vi "Main.vi"(11 "Module Admin":refnum<class "Delacor_lib_QMH_Module Admin.lvclass">) -> ()   [LabVIEW 2024, in "File IO.lvlib"]
doc: "This template is based off of the Queued Message Handler design pattern and the Queued Message Handler project template that ships with LabVIEW.\n\nThe main difference is that the queue is private to this module and communication between modules is performed via Broadcast and Request events.\n\nRequest events are wrapped in public API methods and are handled in the Event Handling Loop (EHL) of this VI. Any module can register for Broadcast events sent by this module. The EHL generates messages based on user interface actions.\n\nThe Message Handling Loop (MHL) processes messages generated by the EHL, or by other messages. The messages are string values, so new messages can be added easily to the Message Cases case structure in the MHL. Each message cluster can also provide an optional value for Message Data, which is a variant that can be converted to whatever message-specific data is required.\n_____\nBased on DQMH Project Template 7.0.1.1316."
uses:
  File IO.lvlib
  <vilib>/Delacor/Delacor QMH/Libraries/Module Admin_class/Delacor_lib_QMH_Module Admin.lvclass
  Module Data--cluster.ctl
  <vilib>/Delacor/Delacor QMH/Libraries/Message Queue_class/Delacor_lib_QMH_Message Queue.lvclass/Delacor_lib_QMH_Message Queue.ctl
  Stop Argument--cluster.ctl
  <vilib>/Delacor/Delacor QMH/Libraries/Module Admin_class/Delacor_lib_QMH_Module Admin.lvclass/Delacor_lib_QMH_Module Admin.ctl
  Start Log Argument--cluster.ctl
  <vilib>/Utility/miscctls.llb/LVPointTypeDef.ctl
  <vilib>/Delacor/Delacor QMH/Libraries/Message Queue_class/Delacor_lib_QMH_Enqueue Message (Single).vi
  <vilib>/Delacor/Delacor QMH/Libraries/Module Admin_class/Delacor_lib_QMH_Get External Launch.vi
  <vilib>/Delacor/Delacor QMH/Libraries/Message Queue_class/Delacor_lib_QMH_Message Queue.lvclass
  Write Argument--cluster.ctl
  <vilib>/Utility/sysdir.llb/System Directory Type.ctl
panel:
  out "File Created":bool=TRUE
  out "error out":errorcluster
  out "Status":string
  in  "Simulate MHL Error":bool
  in  "Simulate EHL Error":bool
  # "Other processes communicate with this Module via its Public API (wrappers for its Request Events).\n\nThis Module communicates with other processes via its Broadcast Events.\nAny process that wants to receive these messages can register for this module's Broadcast events."
  # "This template is for the DQMH framework. See the block diagram for more information on how to use this template."
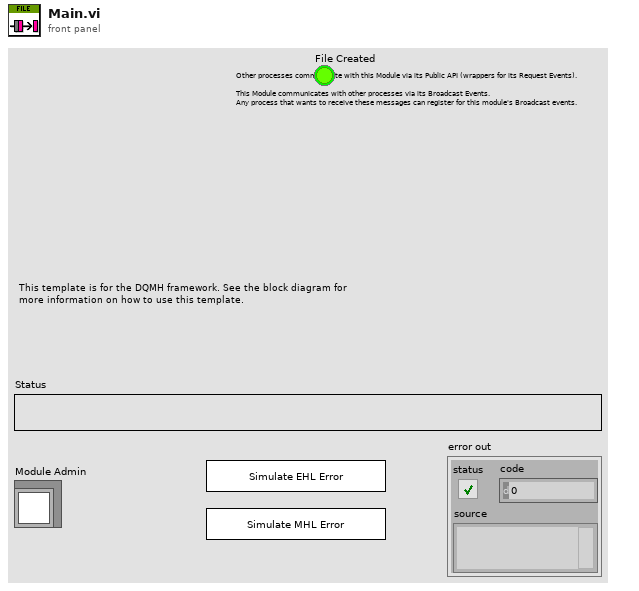
[diagram p1: front panel]
types:
  T1 = typedef "File IO.lvlib/Request Events--cluster.ctl" = cluster{"Stop Module":refnum<user-event>, "Show Panel":refnum<user-event>, "Hide Panel":refnum<user-event>, "Get Module Execution Status":refnum<user-event>, "Show Diagram":refnum<user-event>, "Start Log":refnum<user-event>, "Write":refnum<user-event>}
  T2 = typedef "File IO.lvlib/Module Data--cluster.ctl" = cluster{"Status":string, "LogFilePath":path}
  T3 = enum32{"invalid lock state", "Not Locked", "Locked (No Password)", "Password-protected"}
  T4 = typedef "File IO.lvlib/Stop Argument--cluster.ctl" = cluster{"Origin":string, "Exit via Stop Module Req?":bool, "Wait for Module to stop?":bool}
  T5 = typedef "File IO.lvlib/Start Log Argument--cluster.ctl" = cluster{"Boolean":bool}
  T6 = typedef "File IO.lvlib/Write Argument--cluster.ctl" = cluster{"Write String":string}
  T7 = typedef "LVPointTypeDef.ctl" = cluster{"Horizontal":i16, "Vertical":i16}
  T8 = enum32{"Invalid", "Standard", "Closed", "Hidden", "Minimized", "Maximized"}
  T9 = enum16{"open", "replace", "create", "open or create", "replace or create", "replace or create with confirmation"}
  T10 = typedef "System Directory Type.ctl" = i32
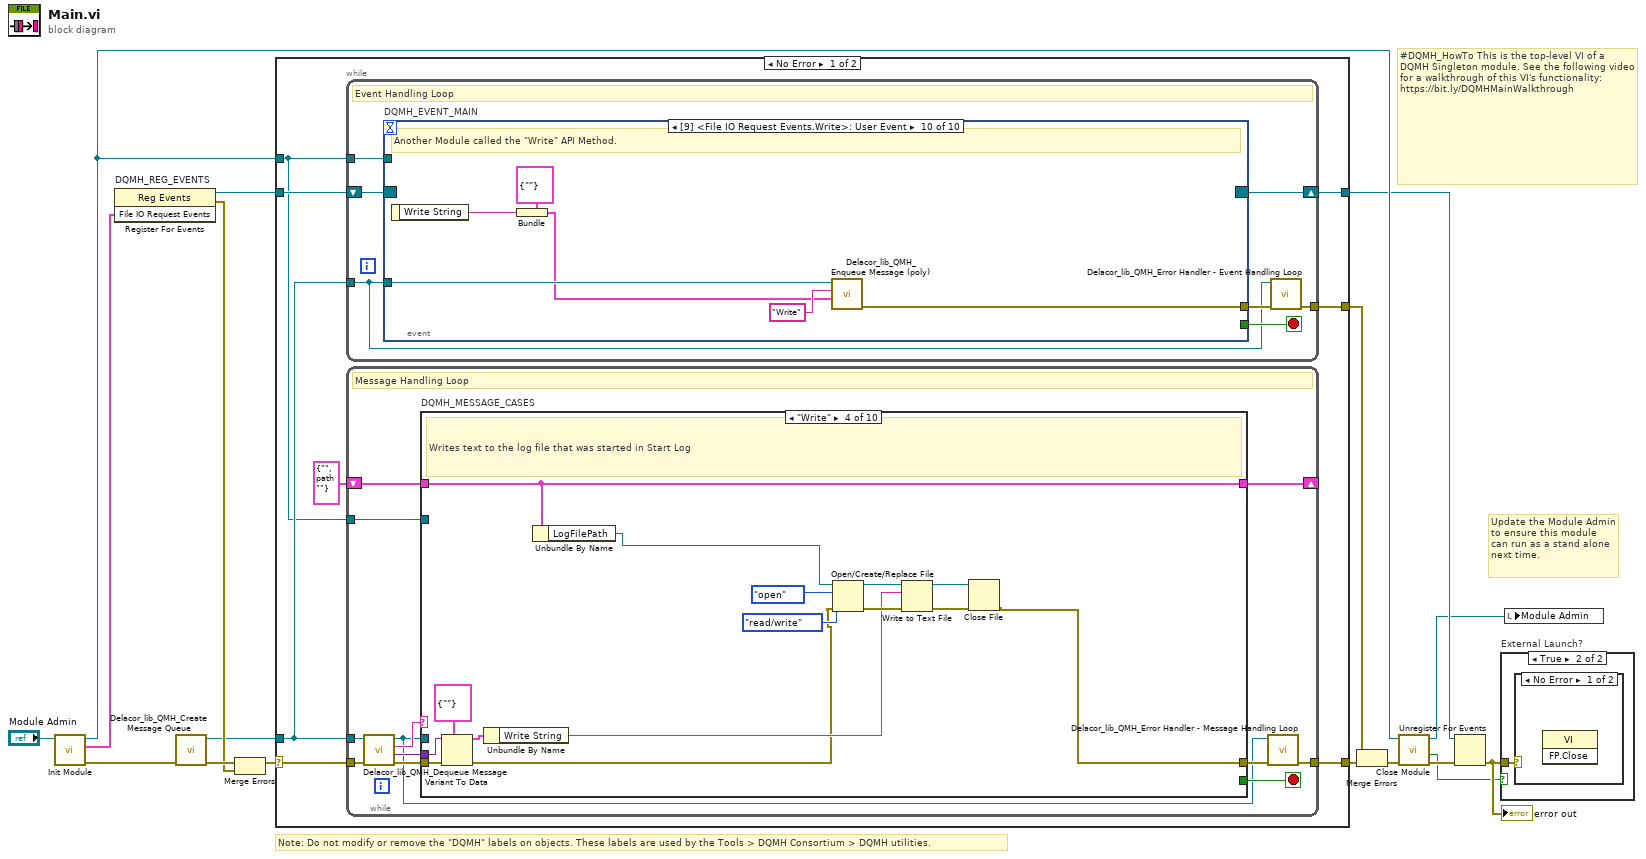
[diagram p0: block diagram]
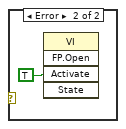
[diagram p3: hidden frame]
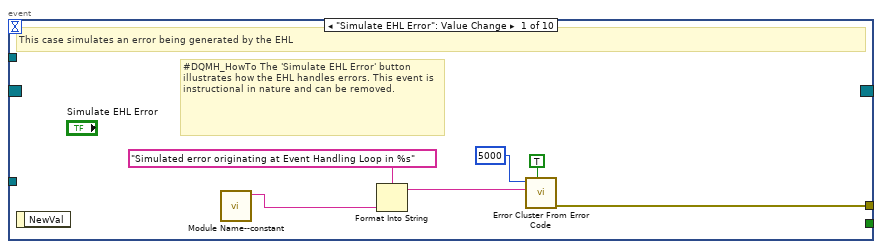
[diagram p4: hidden frame]
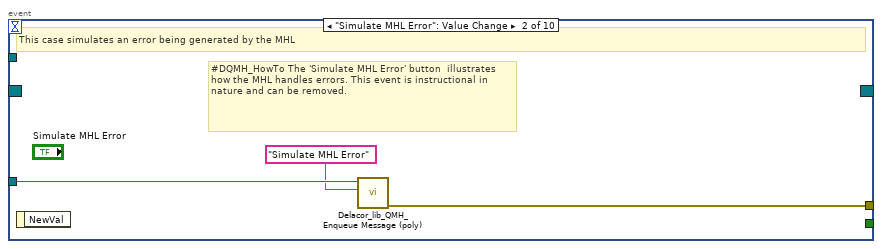
[diagram p5: hidden frame]
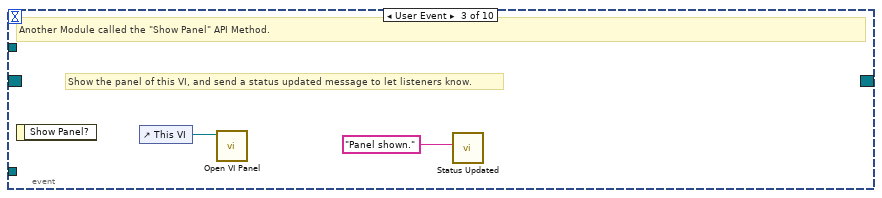
[diagram p6: hidden frame]
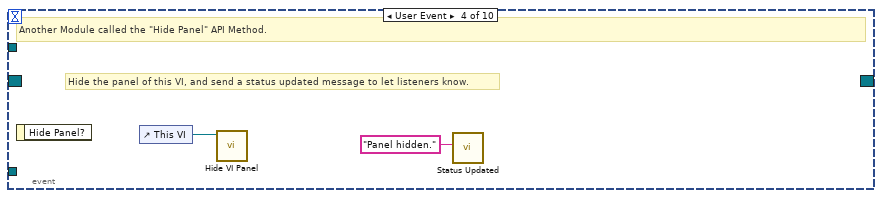
[diagram p7: hidden frame]
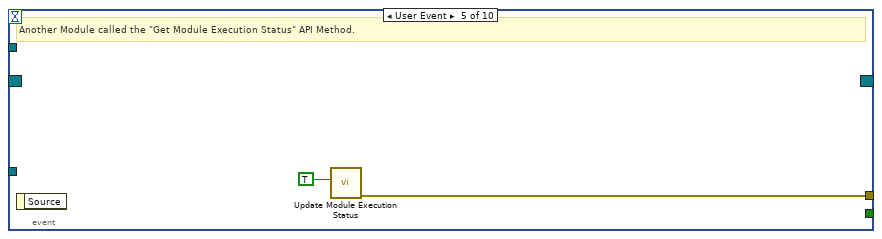
[diagram p8: hidden frame]
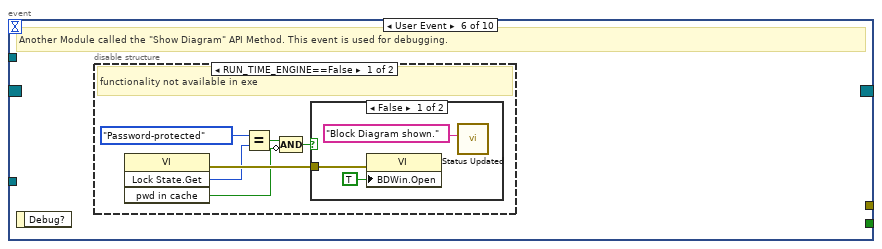
[diagram p9: hidden frame]
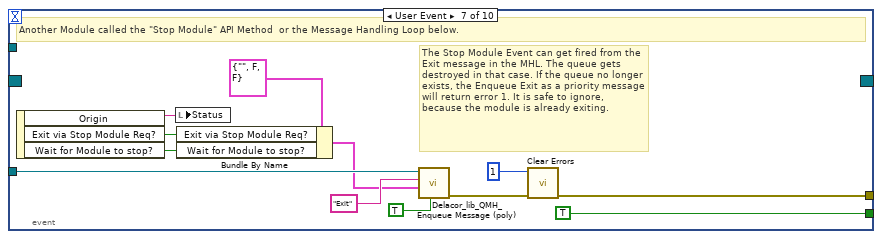
[diagram p12: hidden frame]
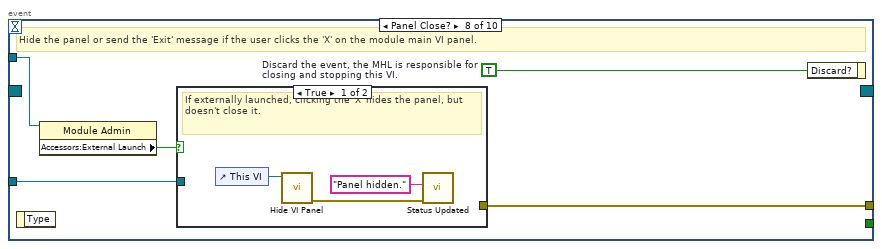
[diagram p13: hidden frame]
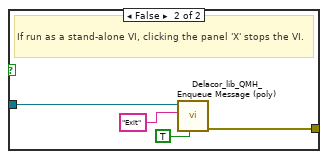
[diagram p14: hidden frame]
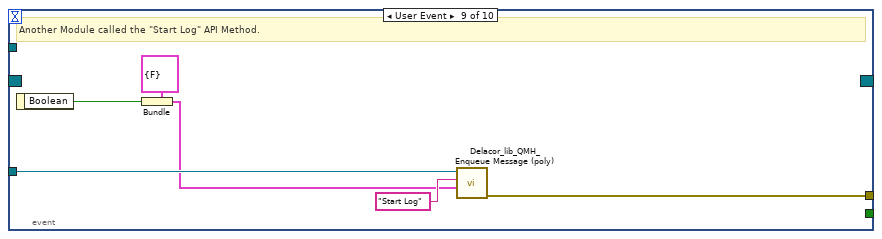
[diagram p15: hidden frame]
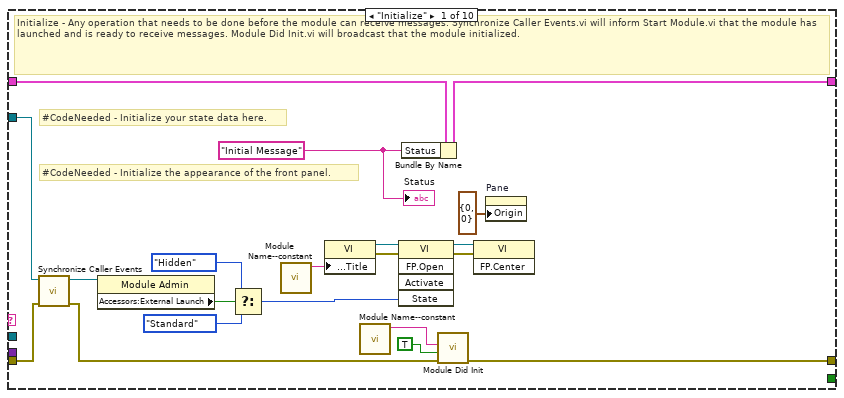
[diagram p16: hidden frame]
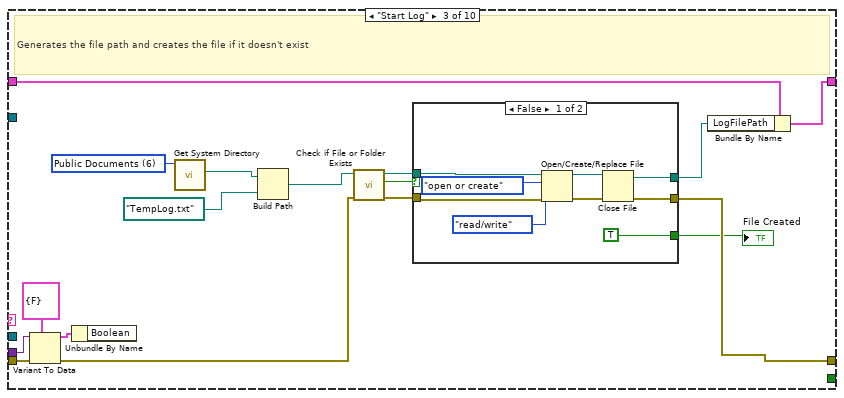
[diagram p18: hidden frame]
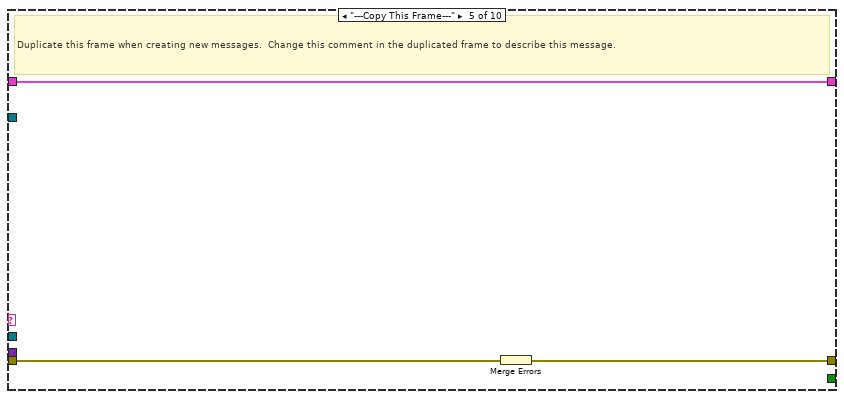
[diagram p20: hidden frame]
diagram:
  # "#DQMH_HowTo This is the top-level VI of a DQMH Singleton module. See the following video for a walkthrough of this VI's functionality: https://bit.ly/DQMHMainWalkthrough"
  # "Note: Do not modify or remove the \"DQMH\" labels on objects. These labels are used by the Tools > DQMH Consortium > DQMH utilities."
  # "Update the Module Admin to ensure this module can run as a stand alone next time."
  n1 = call "Init Module.vi"("Singleton Module Admin in"="Module Admin") -> ("error out"=w16:errorcluster, "File IO Request Events"=w5:T1, "Singleton Module Admin out"=w8:refnum<class "Delacor_lib_QMH_Module Admin.lvclass">)  [unwired: 8 in]
  n2 = register-events "DQMH_REG_EVENTS"(w5) -> (reference out=w6:refnum<event-registration>, error out=w9:errorcluster)  [unwired: 2 in]
  n3 = call <vilib>:"Delacor_lib_QMH_Create Message Queue.vi"("error in"=w16) -> ("error out"=w11:errorcluster, "Message Queue"=w4:refnum<class "Delacor_lib_QMH_Message Queue.lvclass">)  [unwired: 9 in]
  n4 = Merge Errors(w11, w9) -> (w10:errorcluster)
  n5 = case shown="No Error" w10 {
    selector: w10 -> [w23 w233]
    tunnel: [w25 w232] -> w17
    tunnel: [w22 w231] -> w7
    tunnel: w6 -> [w20 w231]
    tunnel: w4 -> [w19 w226]
    tunnel: [w24 _] -> w14
    tunnel: w8 -> [w18 w227]
    frame No Error {
      n6 = while {
        tunnel: w19 -> [w26]
        shift-right: [w29] -> w22
        shift-left: w20 -> [w30]
        tunnel: [w31] -> w24
        tunnel: w18 -> [w27]
        stop <- w28 stop-if-true
        # "Event Handling Loop"
        n7 = event "DQMH_EVENT_MAIN" shown="[9] <File IO Request Events.Write>: User Event" {
          selector: w30 -> [_ _ _ _ _ _ _ _ _ _]
          dyn-events: [_ _ _ _ _ _ _ _ _ _] -> w29
          timeout: _ -> [_ _ _ _ _ _ _ _ _ _]
          tunnel: [_ _ _ _ _ _ TRUE ("Discard?") _ _ _] -> w28
          tunnel: w26 -> [_ w40 _ _ _ _ w64 w71 w86 w92]
          tunnel: [w38 w41 _ _ w47 _ w67 w73 w81 w87] -> w32
          tunnel: w27 -> [_ _ _ _ _ _ _ w70 _ _]
          event "Simulate EHL Error": Value Change {
            # "#DQMH_HowTo The 'Simulate EHL Error' button  illustrates how the EHL handles errors. This event is instructional in nature and can be removed."
            # "This case simulates an error being generated by the EHL"
            n8 = event-data() -> ()  [unwired: 1 in, 1 out]
            n9 = call "Module Name--constant.vi"() -> ("Module Name"=w35:string)  [unwired: 11 in]
            n10 = Format Into String(format string="Simulated error originating at Event Handling Loop in %s", w35) -> (resulting string=w36:string)  [unwired: 2 in, 1 out]
            n11 = call <vilib>:"Error Cluster From Error Code.vi"("show call chain? (False)"=TRUE, "error message (\"\")"=w36, "error code (0)"=5000) -> ("error out"=w38:errorcluster)  [unwired: 6 in]
          }
          event "Simulate MHL Error": Value Change {
            # "#DQMH_HowTo The 'Simulate MHL Error' button  illustrates how the MHL handles errors. This event is instructional in nature and can be removed."
            # "This case simulates an error being generated by the MHL"
            n12 = event-data() -> ()  [unwired: 1 in, 1 out]
            n13 = call-poly <vilib>:"Delacor_lib_QMH_Enqueue Message (poly).vi"("Message"="Simulate MHL Error", "Message Queue in"=w40) -> ("error out"=w41:errorcluster)  [unwired: 8 in, 1 out]
          }
          event User Event {
            # "Show the panel of this VI, and send a status updated message to let listeners know."
            # "Another Module called the \"Show Panel\" API Method."
            n14 = event-data() -> ()  [unwired: 1 in, 1 out]
            n15 = control-ref of="This VI"() -> (w43:refnum<vi>)
            n16 = call "Open VI Panel.vi"("VI"=w43) -> ()  [unwired: 10 in, 1 out]
            n17 = call "Status Updated.vi"("Status"="Panel shown." ("format string")) -> ()  [unwired: 10 in, 1 out]
          }
          event User Event {
            # "Hide the panel of this VI, and send a status updated message to let listeners know."
            # "Another Module called the \"Hide Panel\" API Method."
            n18 = event-data() -> ()  [unwired: 1 in, 1 out]
            n19 = control-ref of="This VI"() -> (w45:refnum<vi>)
            n20 = call "Hide VI Panel.vi"("VI"=w45) -> ()  [unwired: 10 in, 1 out]
            n21 = call "Status Updated.vi"("Status"="Panel hidden." ("format string")) -> ()  [unwired: 10 in, 1 out]
          }
          event User Event {
            # "Another Module called the \"Get Module Execution Status\" API Method."
            n22 = event-data() -> ()  [unwired: 1 in, 1 out]
            n23 = call "Update Module Execution Status.vi"("Running?"=TRUE) -> ("error out"=w47:errorcluster)  [unwired: 10 in]
          }
          event User Event {
            # "Another Module called the \"Show Diagram\" API Method. This event is used for debugging."
            n24 = event-data() -> ()  [unwired: 1 in, 1 out]
            n25 = disable-structure shown="RUN_TIME_ENGINE==False" {
              frame condition #0 (active) {
                # "functionality not available in exe"
                n26 = invoke on="Invoke Node" class="VI" method="Lock State.Get"() -> (error out=w53:errorcluster, "Get Lock State"=w52:T3, "pwd in cache"=w49:bool)  [unwired: 4 in, 1 out]
                n27 = Equal?(x=T3."Password-protected", y=w52) -> (x = y?=w50:bool)
                n28 = Compound Arithmetic op=AND(w50, invert w49) -> (w48:bool)
                n29 = case shown="False" w48 {
                  tunnel: w53 -> [w56 _]
                  frame False {
                    n30 = property on="Property Node" class="VI"(error in=w56, "BDWin.Open"=TRUE ("Block Diagram Window:Open")) -> ()  [unwired: 1 in, 2 out]
                    n31 = call "Status Updated.vi"("Status"="Block Diagram shown." ("format string")) -> ()  [unwired: 10 in, 1 out]
                  }
                  frame True {
                    # "Password-protected VI, and the password is not in the cache. Do not show the diagram."
                  }
                }
              }
              frame condition #1 {
              }
            }
          }
          event User Event {
            # "The Stop Module Event can get fired from the Exit message in the MHL. The queue gets destroyed in that case. If the queue no longer exists, the Enqueue Exit as a priority message will return error 1. It is safe to ignore, because the module is already exiting."
            # "Another Module called the \"Stop Module\" API Method  or the Message Handling Loop below."
            n32 = event-data() -> ("Origin"=w63:string, "Exit via Stop Module Req?"=w59:bool, "Wait for Module to stop?"=w58:bool)  [unwired: 1 in]
            n33 = local write "Status"(w63) -> ()
            n34 = Bundle By Name(cluster=T4 {"Origin"="", "Exit via Stop Module Req?"=FALSE, "Wait for Module to stop?"=FALSE} ("Stop Argument"), "Exit via Stop Module Req?"=w59, "Wait for Module to stop?"=w58) -> (w57:T4)
            n35 = call-poly <vilib>:"Delacor_lib_QMH_Enqueue Message (poly).vi"("Priority Message? (F)"=TRUE, "Message Data"=w57, "Message"="Exit", "Message Queue in"=w64) -> ("error out"=w68:errorcluster)  [unwired: 6 in, 1 out]
            n36 = call <vilib>:"Clear Errors.vi"("error in (no error)"=w68, "specific error code to clear (0: all)"=1) -> ("error out"=w67:errorcluster)  [unwired: 4 in, 1 out]
          }
          event Panel Close? {
            w72 = TRUE  # Discard the event, the MHL is responsible for closing and stopping this VI.
            # "Hide the panel or send the 'Exit' message if the user clicks the 'X' on the module main VI panel."
            n37 = event-data() -> ()  [unwired: 1 in, 1 out]
            n38 = property on="Property Node" class="Module Admin"(reference=w70) -> ("Accessors:External Launch"=w69:bool)  [unwired: 1 in, 2 out]
            n39 = case shown="True" w69 {
              tunnel: w71 -> [_ w79]
              tunnel: [_ w80] -> w73
              frame True {
                # "If externally launched, clicking the 'X' hides the panel, but doesn't close it."
                n40 = control-ref of="This VI"() -> (w76:refnum<vi>)
                n41 = call "Hide VI Panel.vi"("VI"=w76) -> ("error out"=w74:errorcluster)  [unwired: 10 in]
                n42 = call "Status Updated.vi"("error in"=w74, "Status"="Panel hidden." ("format string")) -> ()  [unwired: 9 in, 1 out]
              }
              frame False {
                # "If run as a stand-alone VI, clicking the panel 'X' stops the VI."
                n43 = call-poly <vilib>:"Delacor_lib_QMH_Enqueue Message (poly).vi"("Priority Message? (F)"=TRUE, "Message"="Exit", "Message Queue in"=w79) -> ("error out"=w80:errorcluster)  [unwired: 7 in, 1 out]
              }
            }
            n44 = event-data ("Event Filter Node")("Discard?"=w72) -> ()  [unwired: 1 in, 1 out]
          }
          event User Event {
            # "Another Module called the \"Start Log\" API Method."
            n45 = event-data() -> ("Boolean"=w82:bool)  [unwired: 1 in]
            n46 = Bundle(cluster=T5 {"Boolean"=FALSE} ("Start Log Argument"), "Boolean"=w82) -> (w83:T5)
            n47 = call-poly <vilib>:"Delacor_lib_QMH_Enqueue Message (poly).vi"("Message Data"=w83, "Message"="Start Log", "Message Queue in"=w86) -> ("error out"=w81:errorcluster)  [unwired: 7 in, 1 out]
          }
          event User Event {
            # "Another Module called the \"Write\" API Method."
            n48 = event-data() -> ("Write String"=w88:string)  [unwired: 1 in]
            n49 = Bundle(cluster=T6 {"Write String"=""} ("Write Argument"), "Write String"=w88) -> (w89:T6)
            n50 = call-poly <vilib>:"Delacor_lib_QMH_Enqueue Message (poly).vi"("Message Data"=w89, "Message"="Write", "Message Queue in"=w92) -> ("error out"=w87:errorcluster)  [unwired: 7 in, 1 out]
          }
        }
        n51 = call-dynamic "Delacor_lib_QMH_Error Handler - Event Handling Loop.vi"("error in"=w32, "Message Queue in"=w26) -> ("dup error in"=w31:errorcluster)  [unwired: 8 in, 1 out]
      }
      n52 = while {
        tunnel: w19 -> [w93]
        shift-right: [w101] -> _
        shift-left: T2 {"Status"="", "LogFilePath"=path ""} ("Data Cluster") -> [w102]
        tunnel: w23 -> [w104]
        tunnel: [w96] -> w25
        tunnel: w18 -> [w97]
        stop <- w100 stop-if-true
        # "Message Handling Loop"
        n53 = call-dynamic "Delacor_lib_QMH_Dequeue Message.vi"("error in"=w104, "Message Queue in"=w93) -> ("error out"=w103:errorcluster, "Message Data"=w98:variant, "Message"=w99:string, "Message Queue out"=w94:refnum<class "Delacor_lib_QMH_Message Queue.lvclass">)  [unwired: 6 in]
        n54 = case "DQMH_MESSAGE_CASES" shown="\"Write\"" w99 {
          selector: w99 -> [_ _ _ _ _ _ _ _ _ w221]
          tunnel: w94 -> [_ _ _ _ _ _ _ w187 w209 _]
          tunnel: w103 -> [w122 w126 w143 w169 w172 w174 w183 w194 w215 w224]
          tunnel: [w120 w126 w131 w155 w171 w174 w182 w190 w210 w225] -> w95
          tunnel: w102 -> [w111 w125 w130 w163 w170 w173 w180 w189 w208 w222]
          tunnel: [w110 w125 w129 w163 w170 w173 w180 w189 w208 w222] -> w101
          tunnel: [_ _ _ _ _ _ _ _ w207 _] -> w100
          tunnel: w98 -> [_ _ w142 w168 _ _ _ w188 w206 _]
          tunnel: w97 -> [w112 _ _ _ _ _ _ w186 w201 _]
          frame "Initialize" {
            w106 = "Initial Message" ("Initial Message")
            # "#CodeNeeded - Initialize the appearance of the front panel."
            # "#CodeNeeded - Initialize your state data here."
            # "Initialize - Any operation that needs to be done before the module can receive messages. Synchronize Caller Events.vi will inform Start Module.vi that the module has launched and is ready to receive messages. Module Did Init.vi will broadcast that the module initialized."
            n55 = call "Synchronize Caller Events.vi"("error in"=w122, "Singleton Module Admin in"=w112) -> ("error out"=w121:errorcluster, "Singleton Module Admin out"=w107:refnum<class "Delacor_lib_QMH_Module Admin.lvclass">)  [unwired: 8 in]
            n56 = property on="Property Node" class="Module Admin"(reference=w107) -> ("Accessors:External Launch"=w116:bool)  [unwired: 1 in, 2 out]
            n57 = Select(t=T8."Hidden" ("State"), s=w116, f=T8."Standard" ("State")) -> (s? t:f=w113:T8)
            n58 = call "Module Name--constant.vi"() -> ("Module Name"=w119:string)  [unwired: 11 in]
            n59 = property on="Property Node" class="VI"("Front Panel.Title"=w119) -> (reference out=w118:refnum<vi>, error out=w124:errorcluster)  [unwired: 2 in]
            n60 = call "Module Name--constant.vi"() -> ("Module Name"=w108:string)  [unwired: 11 in]
            n61 = invoke on="Invoke Node" class="VI" method="FP.Open"(reference=w118, error in=w124, "State"=w113) -> (reference out=w117:refnum<vi>, error out=w123:errorcluster)  [unwired: 2 in, 3 out]
            n62 = Bundle By Name(cluster=w111, "Status"=w106) -> (w110:T2)
            n63 = call "Module Did Init.vi"("error in"=w121, "Initialized?"=TRUE, "Origin"=w108) -> ("error out"=w120:errorcluster)  [unwired: 8 in]
            n64 = invoke on="Invoke Node" class="VI" method="FP.Center"(reference=w117, error in=w123) -> ()  [unwired: 1 in, 3 out]
            n65 = property on="Pane" class="Pane"("Origin"=T7 {"Horizontal"=0, "Vertical"=0}) -> ()  [unwired: 2 in, 2 out]
            "Status" <- w106
          }
          frame "---Module Specific---" {
            # "Separator -- The following cases handle messages specific to this Module."
          }
          frame "Start Log" {
            w139 = T10 6 items=["User Home"=0, "User Desktop"=1, "User Documents"=2, "User Application Data"=3, "User Preferences"=4, "User Temporary"=5, "Public Documents"=6, "Public Application Data"=7, "Public Preferences"=8, "Public Cache"=13, "System Core Libraries"=9, "System Installed Libraries"=10, "Application Files"=11, "Boot Volume Root"=12] ("system directory type")
            # "Generates the file path and creates the file if it doesn't exist"
            n66 = Variant To Data(error in=w143, type=T5 {"Boolean"=FALSE} ("Start Log Argument"), Variant=w142) -> (data=w140:T5, error out=w135:errorcluster)
            n67 = Unbundle By Name(w140) -> ()  [unwired: 1 out]
            n68 = call <vilib>:"Get System Directory.vi"("system directory type"=w139) -> ("system directory"=w138:path)  [unwired: 10 in]
            n69 = Build Path(base path=w138, name or relative path=path "TempLog.txt") -> (appended path=w136:path)
            n70 = call <vilib>:"Check if File or Folder Exists.vi"("error in (no error)"=w135, "path"=w136) -> ("error out"=w132:errorcluster, "file or folder exists?"=w133:bool, "dup path"=w134:path)  [unwired: 7 in]
            n71 = case shown="False" w133 {
              tunnel: w134 -> [w152 w153]
              tunnel: w132 -> [w150 w154]
              tunnel: [w148 w154] -> w131
              tunnel: [w145 w153] -> w128
              tunnel: [TRUE _] -> w127
              frame False {
                n72 = Open/Create/Replace File(file path (use dialog)=w152, error in=w150, operation (0:open)=T9."open or create", access (0:read/write)=enum16{"read/write", "read-only", "write-only"}."read/write") -> (refnum out=w151:refnum<file>, error out=w149:errorcluster)  [unwired: 2 in, 1 out]
                n73 = Close File(refnum=w151, error in=w149) -> (path=w145:path, error out=w148:errorcluster)
              }
              frame True {
              }
            }
            "File Created" <- w127
            n74 = Bundle By Name(cluster=w130, "LogFilePath"=w128) -> (w129:T2)
          }
          frame "Write" {
            # "Writes text to the log file that was started in Start Log"
            n75 = Variant To Data(error in=w169, type=T6 {"Write String"=""} ("Write Argument"), Variant=w168) -> (data=w166:T6, error out=w156:errorcluster)
            n76 = Unbundle By Name(w166) -> ("Write String"=w157:string)
            n77 = Unbundle By Name(w163) -> ("LogFilePath"=w162:path)
            n78 = Open/Create/Replace File(file path (use dialog)=w162, error in=w156, operation (0:open)=T9."open", access (0:read/write)=enum16{"read/write", "read-only", "write-only"}."read/write") -> (refnum out=w160:refnum<file>, error out=w161:errorcluster)  [unwired: 2 in, 1 out]
            n79 = Write to Text File(file (use dialog)=w160, text=w157, error in=w161) -> (refnum out=w158:refnum<file>, error out=w159:errorcluster)  [unwired: 1 in, 1 out]
            n80 = Close File(refnum=w158, error in=w159) -> (error out=w155:errorcluster)  [unwired: 1 out]
          }
          frame "---Copy This Frame---" {
            # "Duplicate this frame when creating new messages.  Change this comment in the duplicated frame to describe this message."
            n81 = Merge Errors(w172) -> (w171:errorcluster)
          }
          frame "---Exit and Error Handling---" {
            # "Separator - The following cases handle errors and exit messages."
          }
          frame "Simulate MHL Error" {
            # "#DQMH_HowTo The 'Simulate MHL Error' button  illustrates how the MHL handles errors. This event is instructional in nature and can be removed."
            # "Simulate an error occurring at the MHL"
            n82 = call "Module Name--constant.vi"() -> ("Module Name"=w176:string)  [unwired: 11 in]
            n83 = Format Into String(format string="Simulated error originating at Message Handling Loop in %s", w176) -> (resulting string=w177:string)  [unwired: 2 in, 1 out]
            n84 = call <vilib>:"Error Cluster From Error Code.vi"("show call chain? (False)"=TRUE, "error message (\"\")"=w177, "error code (0)"=5001) -> ("error out"=w181:errorcluster)  [unwired: 6 in]
            n85 = Merge Errors(w183, w181) -> (w182:errorcluster)
          }
          frame "Error" {
            # "#CodeRecommended - If the module is running in standalone mode (External Launch = FALSE), this code will pop up an error dialog and call the 'Exit' message if an error occurs. Add more fine-grained error management here."
            # "Error - Check the error message data and respond accordingly. This message is sent by the \"Error Handler\" VIs at the end of each loop in this application."
            n86 = property on="Property Node" class="Module Admin"(reference=w186) -> ("Accessors:External Launch"=w185:bool)  [unwired: 1 in, 2 out]
            n87 = Variant To Data(error in=w194, type=errorcluster {"status"=FALSE, "code"=0, "source"=""} ("error constant"), Variant=w188) -> (data=w184:errorcluster, error out=w192:errorcluster)
            n88 = local write "error out"(w184) -> ()
            n89 = call "Error Reported.vi"("Error"=w184) -> ()  [unwired: 10 in, 1 out]
            n90 = case shown="False" w185 {
              tunnel: [w199 _] -> w191
              tunnel: w187 -> [w197 _]
              tunnel: w184 -> [w198 _]
              frame False {
                n91 = disable-structure shown="Default" {
                  disable-tunnel: w198 -> [w200 _]
                  frame condition #0 (active) {
                    # "If the module is running standalone, then pop up an error dialog and call the \"Exit\" message."
                    n92 = call <vilib>:"Simple Error Handler.vi"("error in (no error)"=w200) -> ()  [unwired: 4 in, 5 out]
                  }
                  frame condition #1 {
                    # "To prevent the Simple Error Handler VI from being loaded (e.g. when deploying to a Real-Time target), add the Conditional Disable Symbol \"DQMH_Disable_SEH\" to your project and set it to TRUE."
                  }
                }
                n93 = call-poly <vilib>:"Delacor_lib_QMH_Enqueue Message (poly).vi"("Priority Message? (F)"=TRUE, "Message"="Exit", "Message Queue in"=w197) -> ("error out"=w199:errorcluster)  [unwired: 7 in, 1 out]
              }
              frame True {
                # "If the module was launched externally, calling the Error Reported broadcast VI is the only action performed by the \"Error\" message. The module's caller can then process the error appropriately."
              }
            }
            n94 = Merge Errors(w192, w191) -> (w190:errorcluster)
          }
          frame "Exit" {
            w205 = 91  # 91: not all Exit messages will have an argument
            w207 = TRUE  # Stop the VI
            # "Release the message queue reference"
            # "#CodeNeeded - Add any required cleanup code here."
            # "Exit - Exit the application."
            n95 = Variant To Data(error in=w215, type=T4 {"Origin"="", "Exit via Stop Module Req?"=FALSE, "Wait for Module to stop?"=FALSE} ("Stop Argument"), Variant=w206) -> (data=w203:T4, error out=w212:errorcluster)
            n96 = call <vilib>:"Clear Errors.vi"("error in (no error)"=w212, "specific error code to clear (0: all)"=w205) -> ("error out"=w214:errorcluster)  [unwired: 4 in, 1 out]
            n97 = control-ref of="This VI"() -> (w202:refnum<vi>)
            n98 = call-dynamic "Delacor_lib_QMH_Release Message Queue.vi"("error in"=w214, "Message Queue"=w209) -> ("error out"=w213:errorcluster)  [unwired: 9 in]
            n99 = call "Handle Exit.vi"("Stop Argument"=w203, "Admin in"=w201, "VI reference"=w202) -> ("error out"=w211:errorcluster)  [unwired: 7 in, 1 out]
            n100 = Merge Errors(w213, w211) -> (w210:errorcluster)
            n101 = call "Error Reported.vi"("Error"=w210) -> ()  [unwired: 10 in, 1 out]
          }
          frame Default {
            # "'Default' case only runs if there is a message that isn't defined in any of the other cases.  Output a programming error."
            n102 = call "Module Name--constant.vi"() -> ("Module Name"=w220:string)  [unwired: 11 in]
            n103 = Format Into String(format string="The invalid message string \"%s\" was received in the Message Handling Loop for module \"%s\".", w221, w220) -> (resulting string=w216:string)  [unwired: 2 in, 1 out]
            n104 = call <vilib>:"Error Cluster From Error Code.vi"("show call chain? (False)"=TRUE, "error message (\"\")"=w216, "error code (0)"=1) -> ("error out"=w223:errorcluster)  [unwired: 6 in]
            n105 = Merge Errors(w224, w223) -> (w225:errorcluster)
          }
        }
        n106 = call-dynamic "Delacor_lib_QMH_Error Handler - Message Handling Loop.vi"("error in"=w95, "Message Queue in"=w94) -> ("dup error in"=w96:errorcluster)  [unwired: 8 in, 1 out]
      }
    }
    frame Error {
      # "Synchronize Caller Events.vi will inform Start Module.vi that the module has launched and will let the code calling Start Module.vi register for broadcasts and would permit the caller receive the broadcast that an error occurred at launch time."
      n107 = call-dynamic "Delacor_lib_QMH_Release Message Queue.vi"("error in"=w233, "Message Queue"=w226) -> ("error out"=w232:errorcluster)  [unwired: 9 in]
      n108 = call "Synchronize Caller Events.vi"("Singleton Module Admin in"=w227) -> ("error out"=w234:errorcluster)  [unwired: 9 in, 1 out]
      n109 = call "Module Name--constant.vi"() -> ("Module Name"=w230:string)  [unwired: 11 in]
      n110 = Format Into String(format string="An error occurred during initialization. %s is no longer running.", w230) -> (resulting string=w228:string)  [unwired: 2 in, 1 out]
      n111 = Merge Errors(w232, w234) -> (w235:errorcluster)
      n112 = call "Error Reported.vi"("Additional Information"=w228, "Error"=w235) -> ()  [unwired: 9 in, 1 out]
    }
  }
  n113 = Merge Errors(w14, w17) -> (w13:errorcluster)
  n114 = call "Close Module.vi"("error in"=w13, "Module Admin in"=w8) -> ("error out"=w15:errorcluster, "External Launch"=w1:bool, "Module Admin out"=w2:refnum<class "Delacor_lib_QMH_Module Admin.lvclass">)  [unwired: 7 in]
  n115 = Unregister For Events(event registration refnum=w7, error in=w15) -> (error out=w12:errorcluster)
  "error out" <- w12
  n116 = case "External Launch?" shown="True" w1 {
    tunnel: w12 -> [_ w236]
    frame False {
    }
    frame True {
      n117 = case shown="No Error" w236 {
        frame No Error {
          n118 = invoke on="Invoke Node" class="VI" method="FP.Close"() -> ()  [unwired: 3 in, 3 out]
        }
        frame Error {
          n119 = invoke on="Invoke Node" class="VI" method="FP.Open"("Activate"=TRUE ("Activate?")) -> ()  [unwired: 4 in, 5 out]
        }
      }
    }
  }
  n120 = local write "Module Admin"(w2) -> ()
